vi "Send Aquire Data.vi"(7 "Message Priority (Normal)":T1=enum."Normal", 8 "error in (no error)":errorcluster, 10 "Aqusition Time (s)":dbl, 11 "Interlock Q Class in":refnum<class "Interlock Q Class.lvclass">) -> (0 "error out":errorcluster, 3 "Interlock Q Class out":refnum<class "Interlock Q Class.lvclass">)   [LabVIEW 2022 SP3, in "DAQ Process.lvlib" / "Aquire Data Msg.lvclass"]
doc: "This VI sends the message to an actor."
uses:
  Aquire Data Msg.lvclass
  <vilib>/ActorFramework/Message Enqueuer/Message Priority.ctl
  Aquire Data Msg.lvclass/Aquire Data Msg.ctl
  <vilib>/ActorFramework/Message Enqueuer/Message Enqueuer.lvclass/Message Enqueuer.ctl
  <vilib>/ActorFramework/Message Priority Queue/Priority Enqueue.vi
  XY Stage/Process Actor/Process Framework/Interlock Q Class/Interlock Q Class.lvclass
  C:/Program Files/National Instruments/LabVIEW 2022/vi.lib/ActorFramework/Message/Message.lvclass
  C:/XY Stage/IO Monitor/DAQ Actor/DAQ Process Messages/Aquire Data Msg/Aquire Data Msg.lvclass
  <vilib>/ActorFramework/Message Enqueuer/Message Enqueuer.lvclass
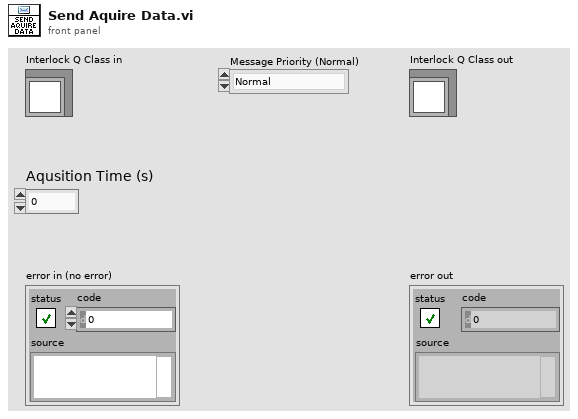
[diagram p1: front panel]
types:
  T1 = typedef "Actor Framework.lvlib/Message Enqueuer.lvclass/Message Priority.ctl" = enum16{"Low", "Normal", "High"}
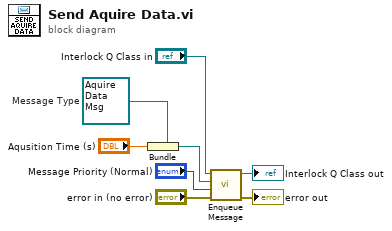
[diagram p0: block diagram]
diagram:
  w8 = refnum<class "Aquire Data Msg.lvclass"> refnum  # Message Type
  n1 = Bundle(cluster=w8, "Aqusition Time (s)") -> (w3:refnum<class "Aquire Data Msg.lvclass">)
  n2 = call-dynamic "Enqueue Message.vi"("error in (no error)"="error in (no error)", "Message Priority (Normal)"="Message Priority (Normal)", "Message"=w3, "Interlock Q Class in"="Interlock Q Class in") -> ("error out"=→"error out":errorcluster, "Interlock Q Class out"=→"Interlock Q Class out":refnum<class "Interlock Q Class.lvclass">)  [unwired: 6 in]
